vi "Find_center_distance.vi"() -> ()   [LabVIEW 2016]
uses:
  Classes/Controllers/Motion/Copy of Motion Folder/Motion.lvclass
  Classes/Controllers/Camera/Copy of Controller Folder/Controller.lvclass
panel:
  in  "Stop":bool
  in  "DO measurement":bool=TRUE
  out "sample size":dbl[](array[numeric])
  out "Sum 2":dbl[](array[numeric])
  out "Sum 1":dbl[](array[numeric])
  out "r-phi":dbl[](array[numeric])
  out "CENTER of two points":dbl[](array[numeric]) format="%#_10g"
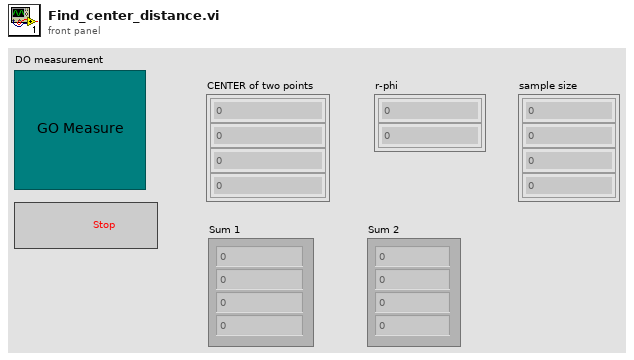
[diagram p1: front panel]
types:
  T1 = typedef "Controller.lvclass/Controllers.ctl" = cluster{"Copy of Motion.lvclass":refnum<class "Motion.lvclass">, "Copy of I-O.lvclass":refnum<class "I-O.lvclass">, "Copy of Dispenser.lvclass":refnum<class "Dispenser.lvclass">}
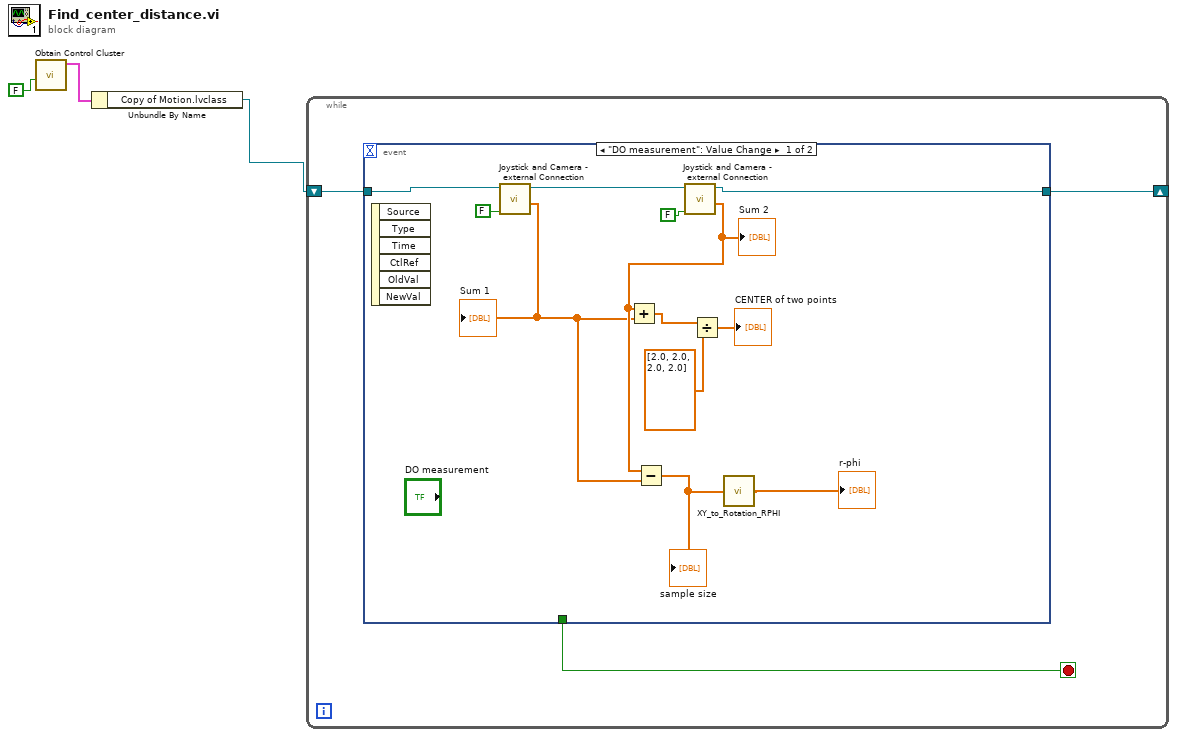
[diagram p0: block diagram]
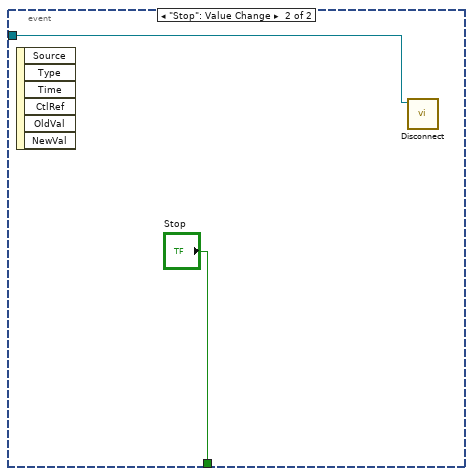
[diagram p2: hidden frame]
diagram:
  n1 = call "Obtain Control Cluster.vi"("I/O"=FALSE) -> ("Control Out"=w3:T1)  [unwired: 10 in]
  n2 = Unbundle By Name(w3) -> ("Copy of Motion.lvclass"=w1:refnum<class "Motion.lvclass">)
  n3 = while {
    shift-right: [w5] -> _
    shift-left: w1 -> [w6]
    stop <- w4 stop-if-true
    n4 = event shown="[0] \"DO measurement\": Value Change" {
      selector: _ -> [_ _]
      dyn-events: _ -> [_ _]
      timeout: _ -> [_ _]
      tunnel: w6 -> [w12 w20]
      tunnel: [w11 _] -> w5
      tunnel: [_ "Stop"] -> w4
      event "DO measurement": Value Change {
        n5 = event-data() -> ()  [unwired: 1 in, 6 out]
        n6 = call "Joystick and Camera - external Connection.vi"("Motion in"=w12, "Inital GO"=FALSE) -> ("Motion out"=w16:refnum<class "Motion.lvclass">, "Gantry"=w7:dbl[])  [unwired: 5 in, 2 out]
        "Sum 1" <- w7
        n7 = call "Joystick and Camera - external Connection.vi"("Motion in"=w16, "Inital GO"=FALSE) -> ("Motion out"=w11:refnum<class "Motion.lvclass">, "Gantry"=w8:dbl[])  [unwired: 5 in, 2 out]
        "Sum 2" <- w8
        n8 = Add(x=w8, y=w7) -> (x+y=w15:dbl[])
        n9 = Subtract(x=w8, y=w7) -> (x-y=w9:dbl[])
        "sample size" <- w9
        n10 = Divide(x=w15, y=dbl[] [2.0, 2.0, 2.0, 2.0]) -> (x/y=→"CENTER of two points":dbl[])
        n11 = call "XY_to_Rotation_RPHI.vi"("X-Y"=w9) -> ("r-phi"=→"r-phi":dbl[])
      }
      event "Stop": Value Change {
        n12 = event-data() -> ()  [unwired: 1 in, 6 out]
        n13 = call-dynamic "Disconnect.vi"("Controller in"=w20) -> ()  [unwired: 9 in, 1 out]
      }
    }
  }
